vi "Resize Compare Data.vi"(10 "Size":i32, 11 "Compares in":cluster{"Color":u32, "Info 2":T1}[](array[cluster]) {"Info 2"."Internal Resistance" min=0.0 step=0.005 format="%#_13g"; "Info 2"."Battery Voltage" min=6.0 format="%#_13g"; "Info 2"."Total Mass" min=0.0 step=2.2679618500000003; "Info 2"."Total Amps" min=0.0 step=20.0 format="%#_13g"; "Info 2"."Ratio" min=0.005 step=0.01; "Info 2"."Motor Count" min=2 step=2}) -> (3 "Compares out":cluster{"Color":u32, "Info 2":T1}[](array[cluster]) {"Info 2"."Internal Resistance" min=0.0 step=0.005 format="%#_13g"; "Info 2"."Battery Voltage" min=6.0 format="%#_13g"; "Info 2"."Total Mass" min=0.0 step=2.2679618500000003; "Info 2"."Total Amps" min=0.0 step=20.0 format="%#_13g"; "Info 2"."Ratio" min=0.005 step=0.01; "Info 2"."Motor Count" min=2 step=2})   [LabVIEW 2020]
uses:
  Robot Compare Info.ctl
  Motor Type.ctl
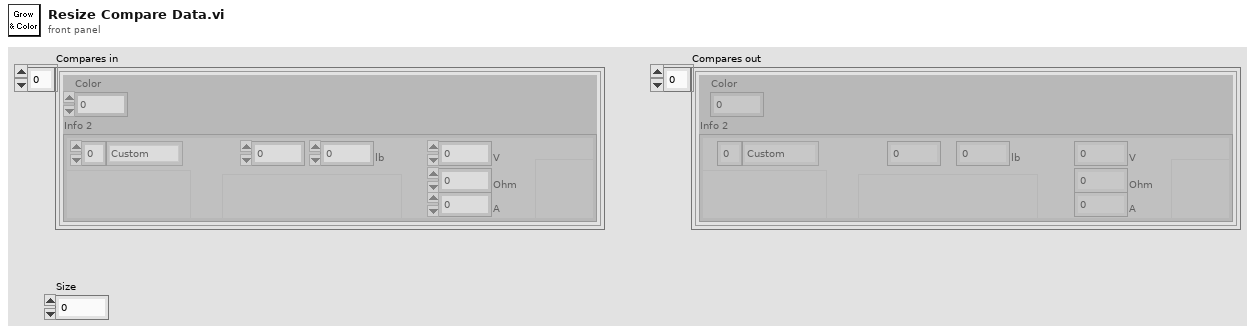
[diagram p1: front panel]
types:
  T1 = typedef "Robot Compare Info.ctl" = cluster{"Motor Count":i32, "Motor Type":T2, "Ratio":dbl, "Total Mass":dbl[unit], "Battery Voltage":dbl[unit], "Internal Resistance":dbl[unit], "Total Amps":dbl[unit]}
  T2 = typedef "Motor Type.ctl" = enum16{"Custom", "775 pro", "CIM", "miniCIM", "Neo", "Neo 550", "Falcon 500"}
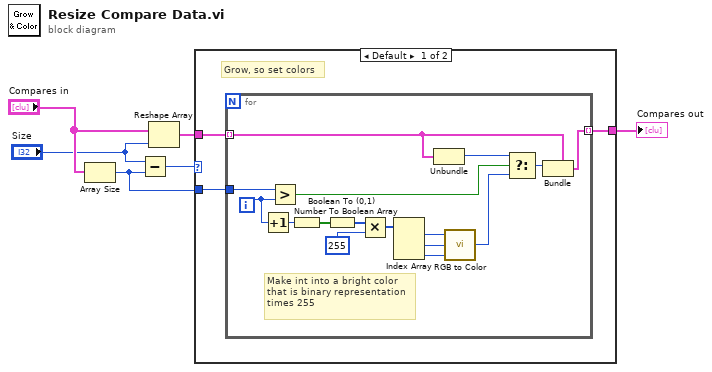
[diagram p0: block diagram]
diagram:
  n1 = Array Size(array="Compares in") -> (size(s)=w1:i32)
  n2 = Subtract(x="Size", y=w1) -> (x-y=w4:i32)
  n3 = Reshape Array("Compares in", "Size") -> (w3:cluster{"Color":u32, "Info 2":T1}[])
  n4 = case shown="Default" w4 {
    tunnel: w3 -> [w9 w26]
    tunnel: [w8 w26] -> w2
    tunnel: w1 -> [w7 _]
    frame Default {
      # "Grow, so set colors"
      n5 = for {
        tunnel: w9 -> [w10] mode=indexing
        tunnel: [w25] -> w8 mode=indexing
        tunnel: w7 -> [w24]
        i -> [w20]
        # "Make int into a bright color\nthat is binary representation\ntimes 255"
        n6 = Increment(x=w20) -> (x+1=w19:i32)
        n7 = Greater?(x=w24, y=w20) -> (0:w23:bool)
        n8 = Number To Boolean Array(number=w19) -> (Boolean array=w18:bool[])
        n9 = Boolean To (0,1)(Boolean=w18) -> (0, 1=w16:i16[])
        n10 = Multiply(x=w16, y=u8 255) -> (x*y=w15:i16[])
        n11 = Index Array(array=w15) -> (element #1=w14:i16, element #2=w13:i16, element #3=w12:i16)  [unwired: 3 in]
        n12 = Unbundle(w10) -> ("Color"=w22:u32)  [unwired: 1 out]
        n13 = call <vilib>:"RGB to Color.vi"("B"=w12, "G"=w13, "R"=w14) -> ("Color"=w11:u32)
        n14 = Select(t=w22, s=w23, f=w11) -> (s? t:f=w21:u32)
        n15 = Bundle(cluster=w10, "Color"=w21) -> (w25:cluster{"Color":u32, "Info 2":T1})  [unwired: 1 in]
      }
    }
    frame ..0 {
      # "Same or shrinking"
    }
  }
  "Compares out" <- w2
